vi "Set Result Tree Icons.vi"(8 "error in (no error)":errorcluster, 11 "Tree Refnum":refnum<vi>) -> (0 "error out":errorcluster)   [LabVIEW 2017, in "Test Explorer.lvlib"]
uses:
  Test Explorer.lvlib
  <vilib>/picture/picture.llb/imagedata.ctl
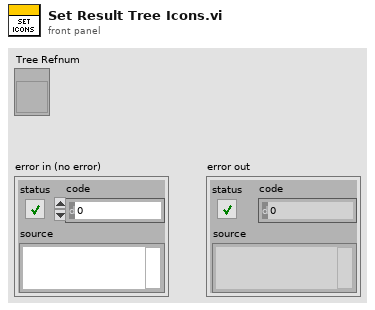
[diagram p1: front panel]
types:
  T1 = typedef "imagedata.ctl" = cluster{"image type":i32, "image depth":i32, "image":u8[], "mask":u8[], "colors":u32[], "Rectangle":cluster{"left":i16, "top":i16, "right":i16, "bottom":i16}}
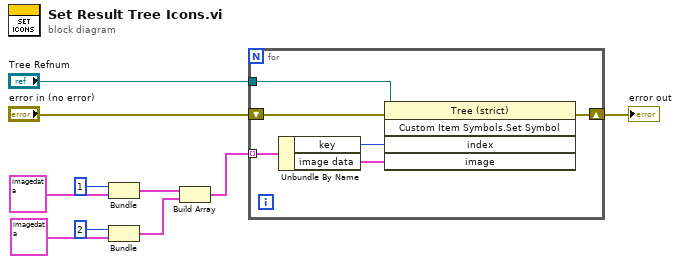
[diagram p0: block diagram]
diagram:
  n1 = Bundle("key"=1, "image data"=T1 {"image type"=0, "image depth"=32, "image"=array[1024 elements], "mask"=[7, 224, 15, 240, 63, 252, 63, 252, 127, 254, 255, 255, 255, 255, 255, 255, 255, 255, 255, 255, 255, 255, 127, 254, 63, 252, 63, 252, 15, 240, 7, 224], "colors"=[], "Rectangle"={"left"=0, "top"=0, "right"=16, "bottom"=16}}) -> (w3:cluster{"key":i32, "image data":T1})  [unwired: 1 in]
  n2 = Bundle("key"=2, "image data"=T1 {"image type"=0, "image depth"=32, "image"=array[1024 elements], "mask"=[7, 224, 15, 240, 63, 252, 63, 252, 127, 254, 255, 255, 255, 255, 255, 255, 255, 255, 255, 255, 255, 255, 127, 254, 63, 252, 63, 252, 15, 240, 7, 224], "colors"=[], "Rectangle"={"left"=0, "top"=0, "right"=16, "bottom"=16}}) -> (w2:cluster{"key":i32, "image data":T1})  [unwired: 1 in]
  n3 = Build Array(w3, w2) -> (w1:cluster{"key":i32, "image data":T1}[])
  n4 = for {
    tunnel: "Tree Refnum" -> [w16]
    tunnel: w1 -> [w15] mode=indexing
    shift-right: [w11] -> w8
    shift-left: "error in (no error)" -> [w12]
    n5 = Unbundle By Name(w15) -> ("key"=w14:i32, "image data"=w13:T1)
    n6 = invoke class="Tree (strict)" method="Custom Item Symbols.Set Symbol"(reference=w16, error in=w12, "index"=w14, "image"=w13) -> (error out=w11:errorcluster)  [unwired: 1 in, 4 out]
  }
  "error out" <- w8
